vi "E01_Tipo de datos.vi"() -> ()   [LabVIEW 2026]
panel:
  out "Array":dbl[](array[numeric])
  out "Cluster":cluster{"Numeric":dbl, "Numeric 2":dbl}
  out "String":string
  out "Numeric 4":dbl
  out "Numeric 3":i32
  out "Numeric 2":i32
  out "Numeric":dbl
  out "Tank":dbl(slide) scale=0.0..10.0
  in  "Entero":i32
  in  "Double":dbl
  out "LED_03":bool
  in  "Control":bool
  out "LED_02":bool
  out "LED_01":bool
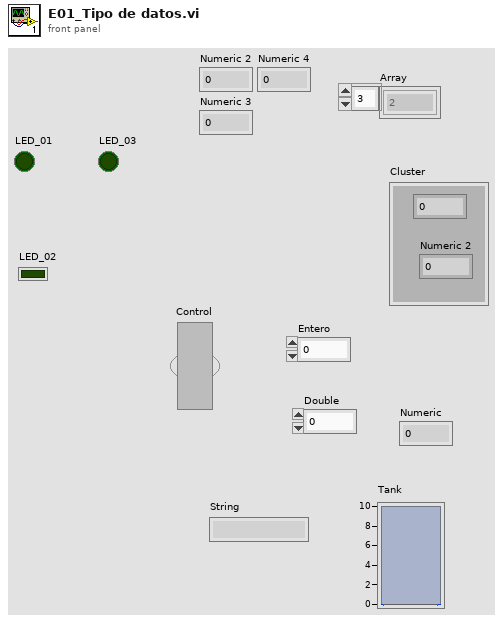
[diagram p1: front panel]
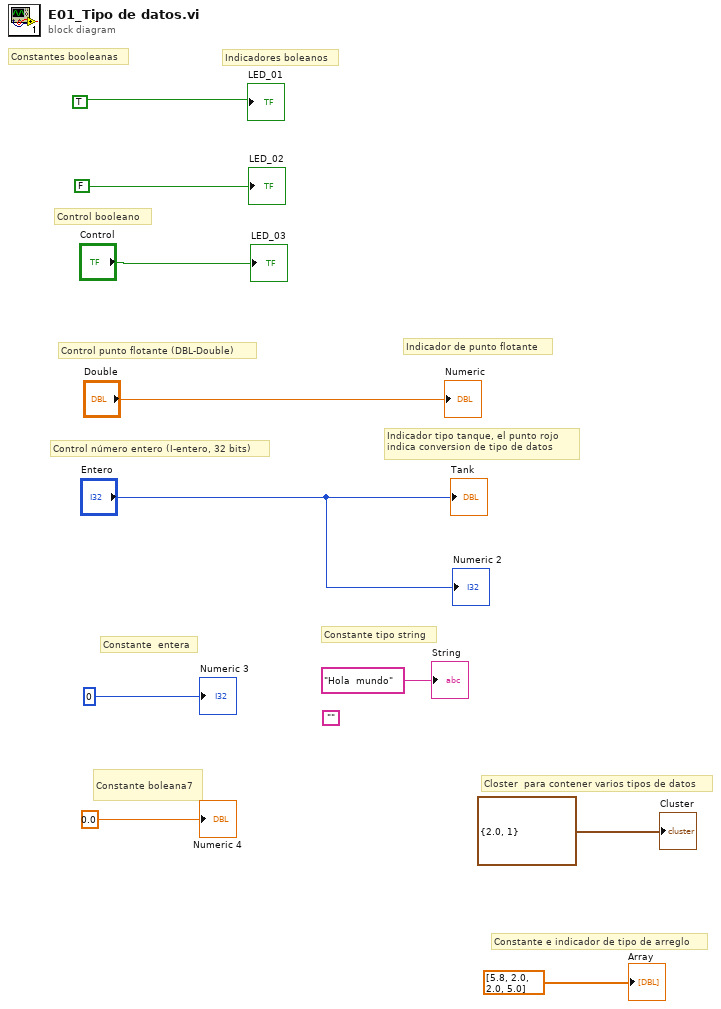
[diagram p0: block diagram]
diagram:
  (unwired) ""
  # "Constante e indicador de tipo de arreglo"
  # "Closter  para contener varios tipos de datos"
  # "Constante tipo string"
  # "Constante boleana7"
  # "Constante  entera"
  # "Indicador de punto flotante"
  # "Indicador tipo tanque, el punto rojo \nindica conversion de tipo de datos"
  # "Control número entero (I-entero, 32 bits)"
  # "Control punto flotante (DBL-Double)"
  # "Control booleano"
  # "Constantes booleanas"
  # "Indicadores boleanos"
  "LED_01" <- TRUE
  "LED_02" <- FALSE
  "LED_03" <- "Control"
  "Tank" <- "Entero"
  "Numeric" <- "Double"
  "Numeric 2" <- "Entero"
  "Numeric 3" <- 0
  "Numeric 4" <- 0.0
  "String" <- "Hola  mundo"
  "Cluster" <- cluster{dbl, i32} {2.0, 1}
  "Array" <- dbl[] [5.8, 2.0, 2.0, 5.0]
